vi "getIgorConversion.vi"(0 "index":i32(ring) items=["ZLVDT sensor", "ZLVDT offset", "XLVDT sensor", "XLVDT offset", "YLVDT sensor", "YLVDT offset", "DEFL"]) -> (1 "Result":dbl format="%#_5p", 2 "error out":errorcluster)   [LabVIEW 2013]
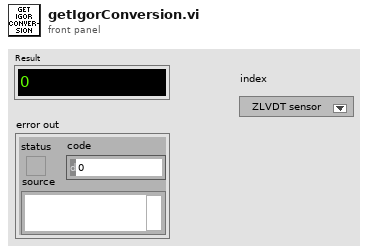
[diagram p1: front panel]
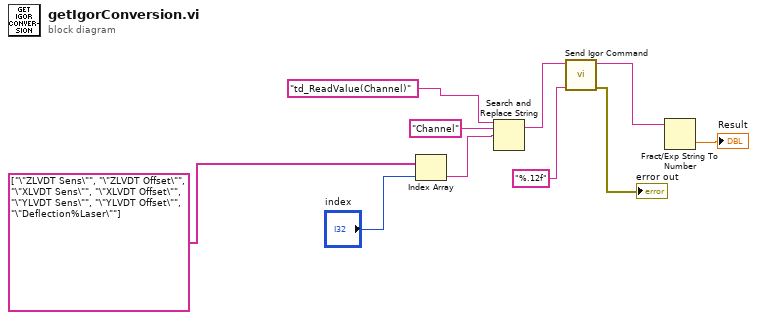
[diagram p0: block diagram]
diagram:
  n1 = Index Array(array=string[] ["\"ZLVDT Sens\"", "\"ZLVDT Offset\"", "\"XLVDT Sens\"", "\"XLVDT Offset\"", "\"YLVDT Sens\"", "\"YLVDT Offset\"", "\"Deflection%Laser\""], index="index") -> (element=w9:string)
  n2 = Search and Replace String(input string="td_ReadValue(Channel)", search string="Channel", replace string=w9) -> (result string=w4:string)  [unwired: 1 in, 7 out]
  n3 = call <vilib>:"Send Igor Command.vi"("Command"=w4, "Expected output Format"="%.12f") -> ("results"=w3:string, "error out"=→"error out":errorcluster)  [unwired: 6 in, 1 out]
  n4 = Fract/Exp String To Number(string=w3) -> (number=→"Result":dbl)  [unwired: 4 out]
